vi "Motor Control Message Loop.vi"(8 "error in (no error)":errorcluster, 10 "Data Queue":refnum<queue>, 11 "Message Queues":T1) -> (0 "error out":errorcluster)   [LabVIEW 2016, in "Message Loop Template.lvlib"]
doc: "The message loop subVI to handle messages pertaining to logging data."
uses:
  Message Loop Template.lvlib
  support/Message Queue/All Message Queues.ctl
  support/Message Queue/Message Cluster.ctl
  Motor Control State.ctl
  Motor Control Config.ctl
  Speed and Duration.ctl
  support/Message Queue/Enqueue Message (Single).vi
  <vilib>/Utility/error.llb/Error Cluster From Error Code.vi
  <vilib>/ErrorRing/Error Ring.xnode
  support/Message Queue/Message Queue.lvlib
panel:
  out "Actual Sample Rate":dbl=1000.0 format="%0.2f"
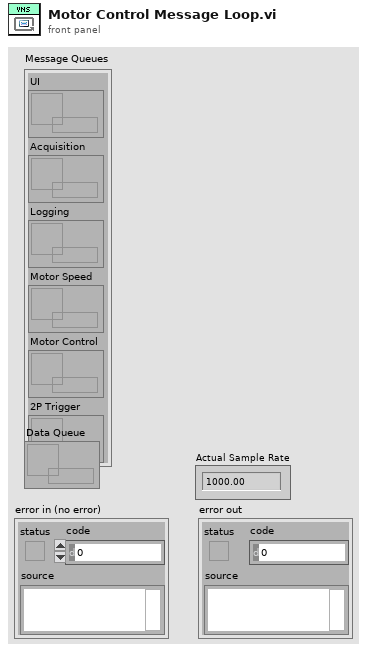
[diagram p1: front panel]
types:
  T1 = typedef "Message Queue.lvlib/All Message Queues.ctl" = cluster{"UI":refnum<queue>, "Acquisition":refnum<queue>, "Logging":refnum<queue>, "Motor Speed":refnum<queue>, "Motor Control":refnum<queue>, "2P Trigger":refnum<queue>}
  T2 = typedef "Message Loop Template.lvlib/Motor Control State.ctl" = enum16{"Idle", "Running"}
  T3 = typedef "Message Loop Template.lvlib/Motor Control Config.ctl" = cluster{"Speed and Duration":T4[]}
  T4 = typedef "Message Loop Template.lvlib/Speed and Duration.ctl" = cluster{"Speed (%)":dbl, "Duration (sec)":dbl}
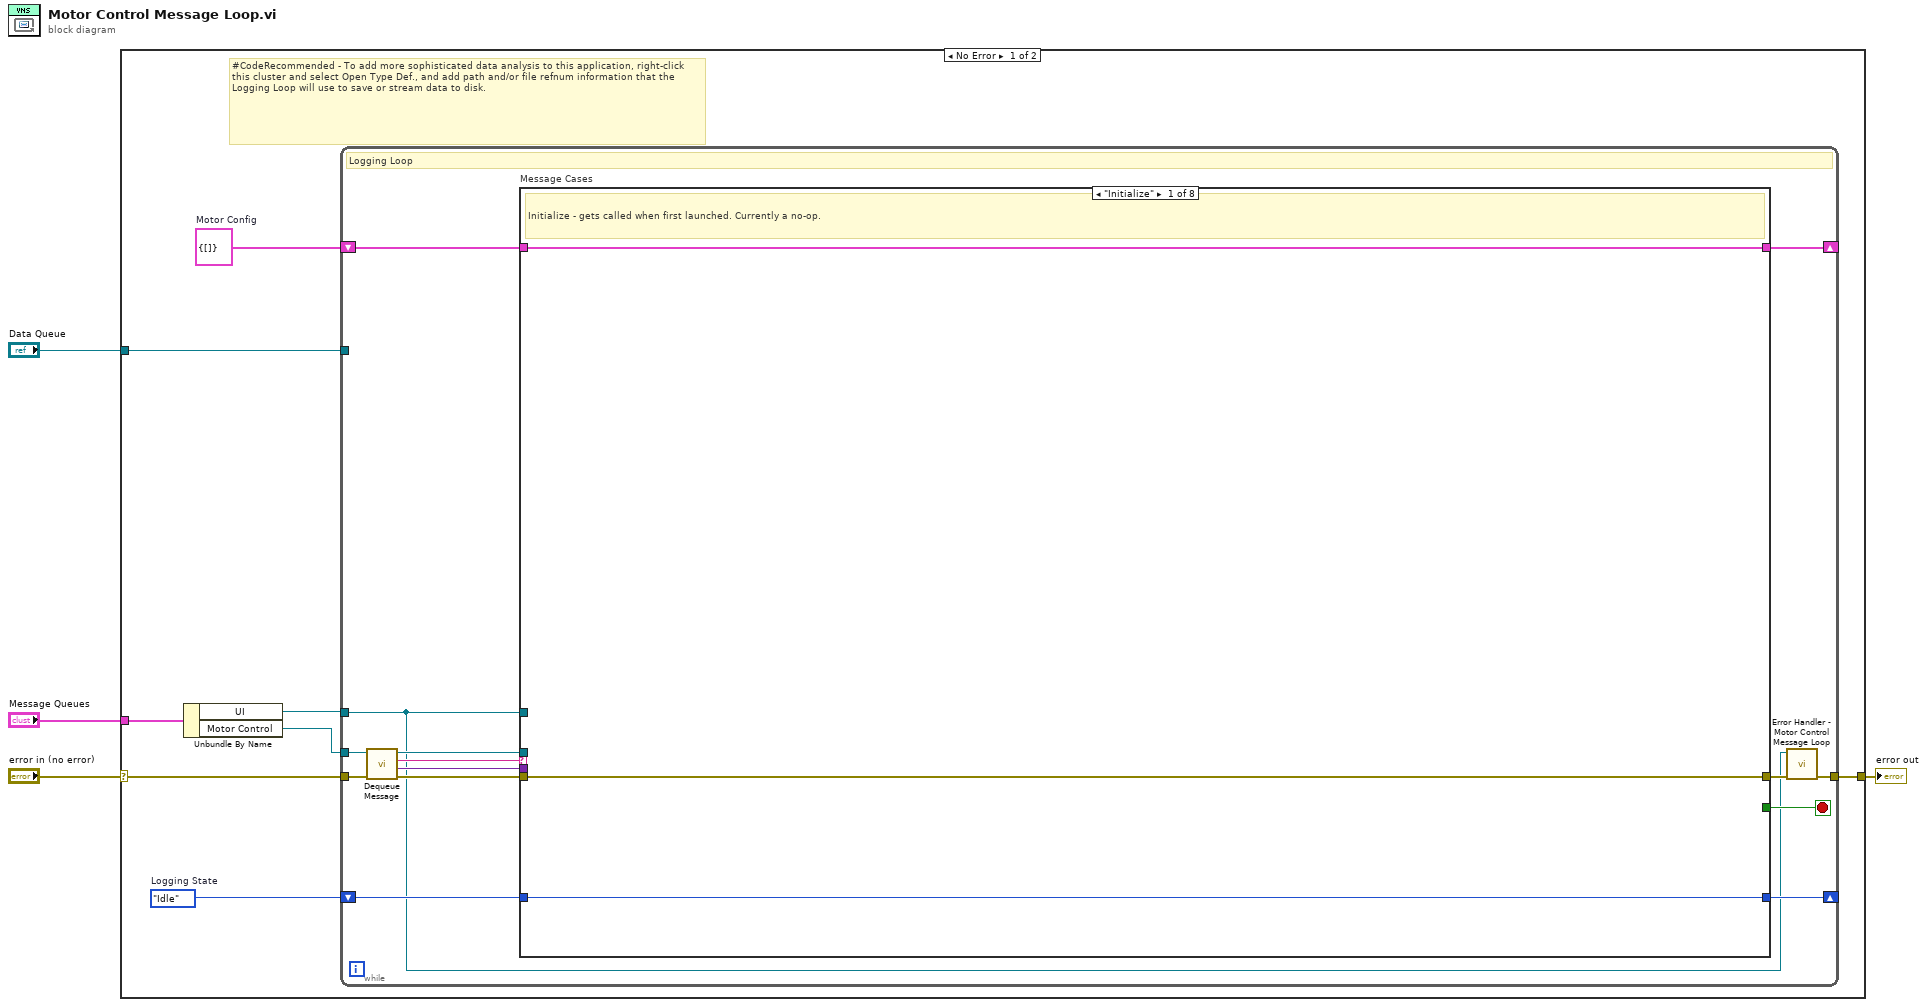
[diagram p0: block diagram]
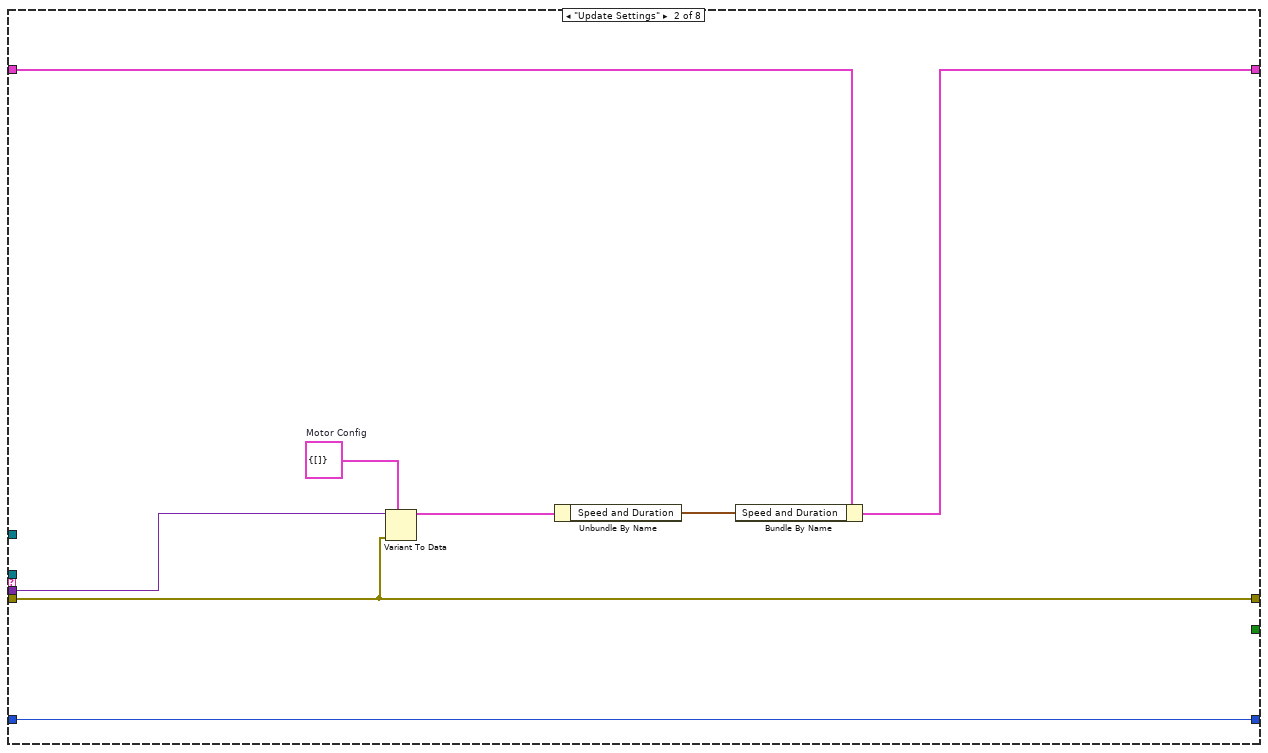
[diagram p2: hidden frame]
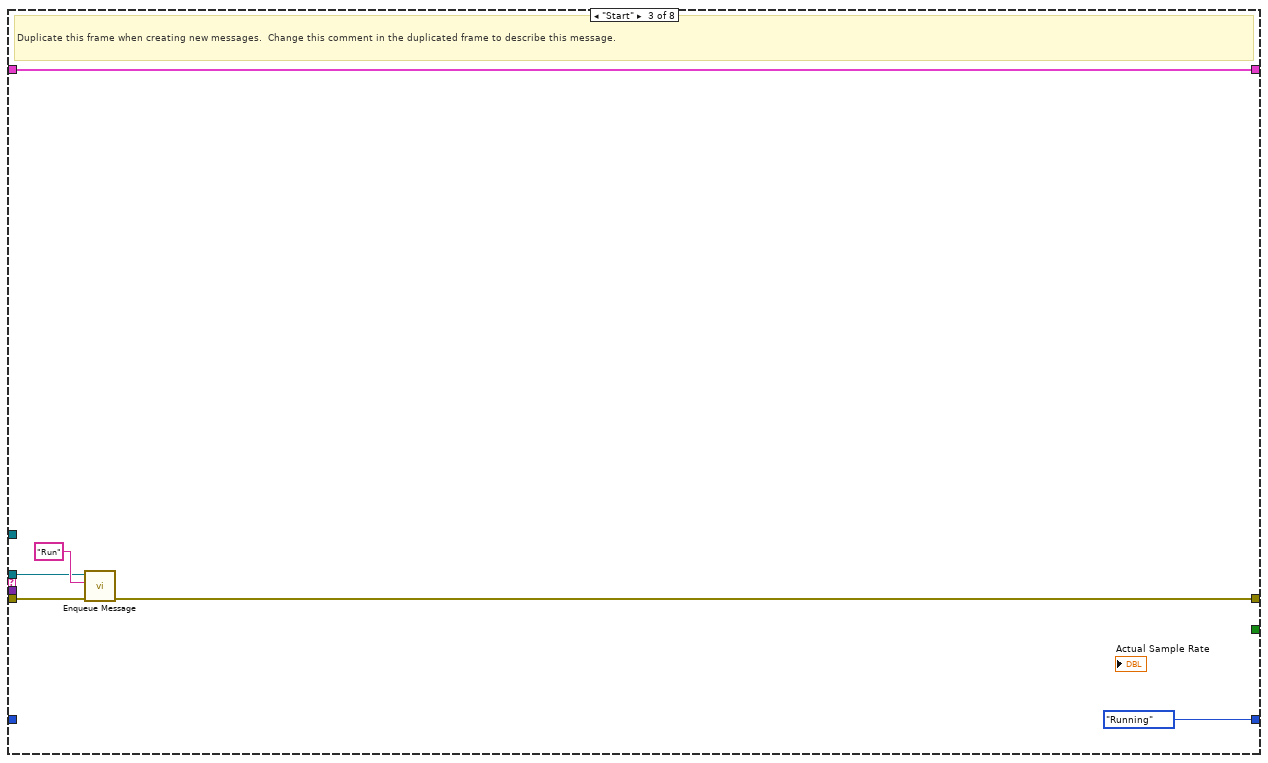
[diagram p3: hidden frame]
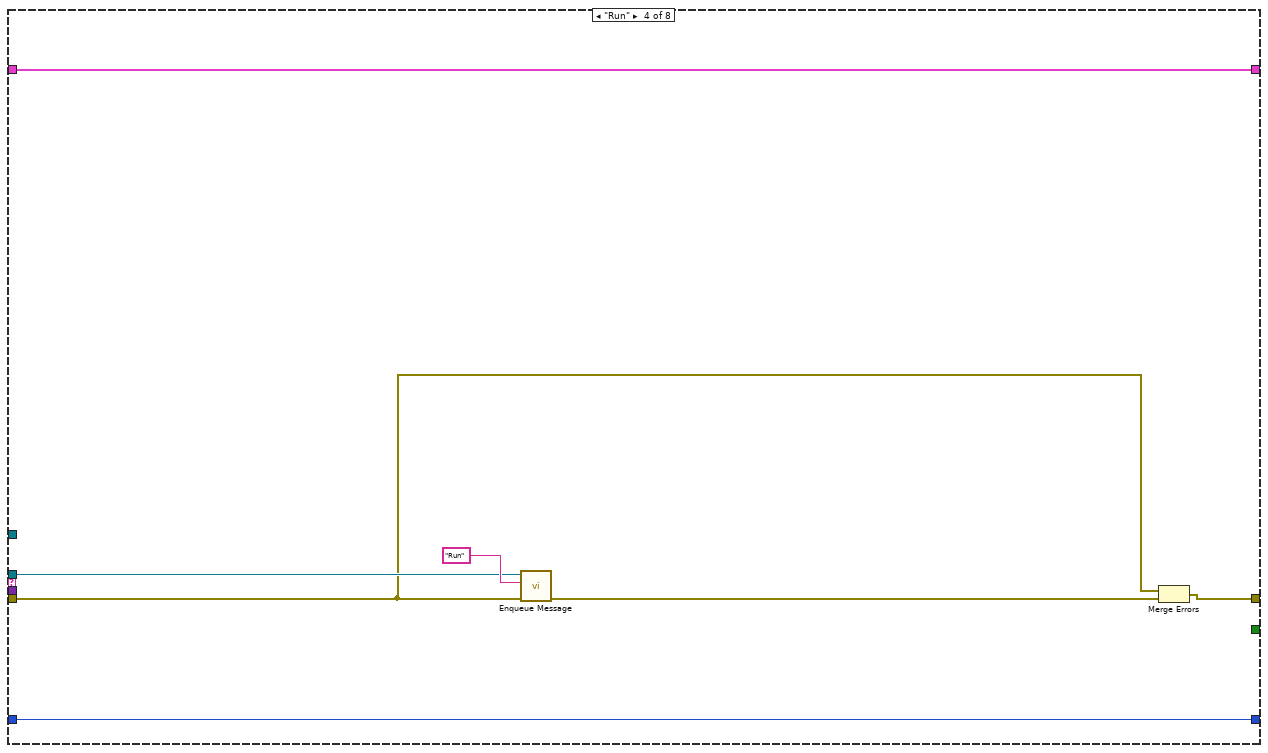
[diagram p4: hidden frame]
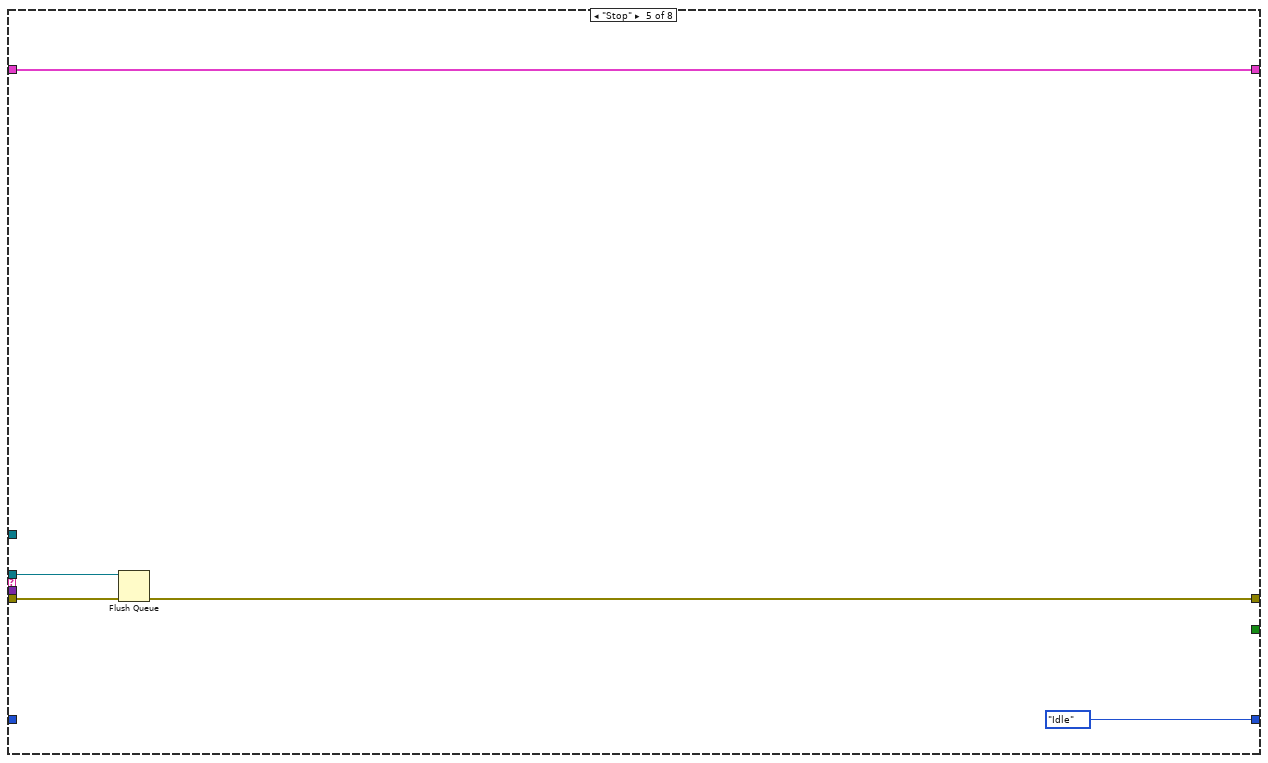
[diagram p5: hidden frame]
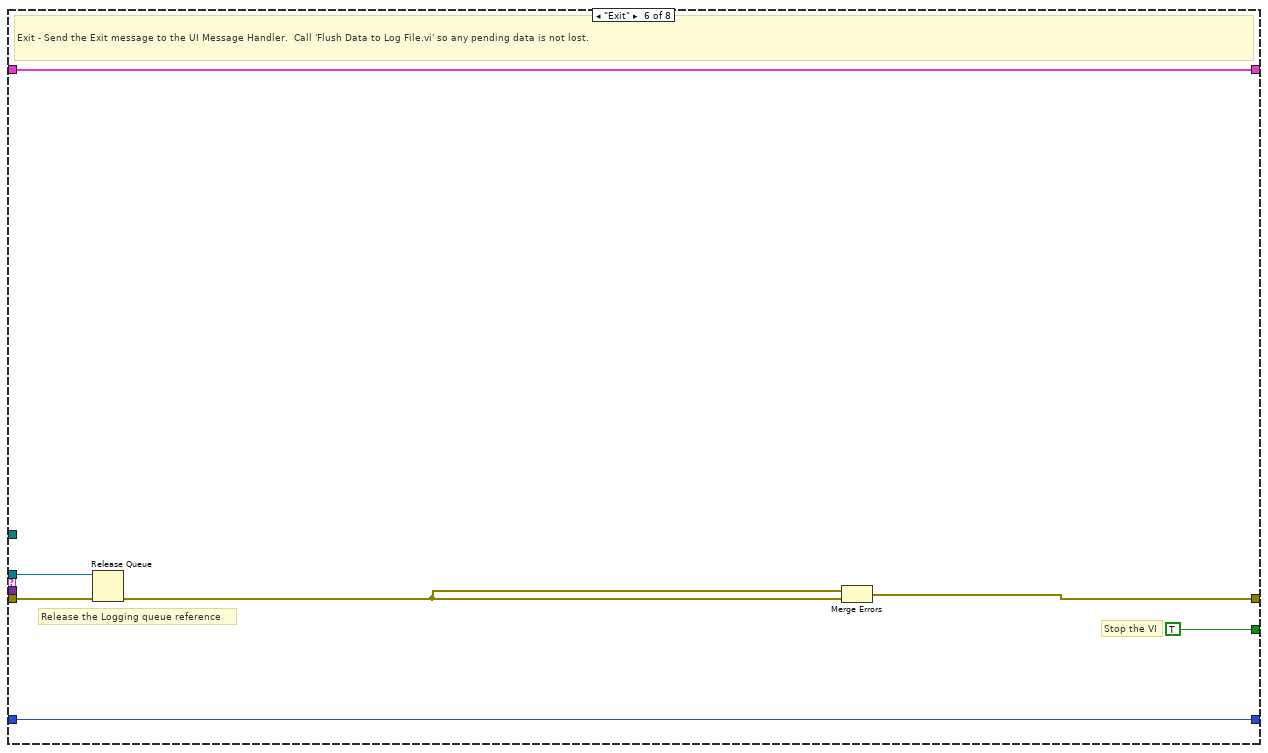
[diagram p6: hidden frame]
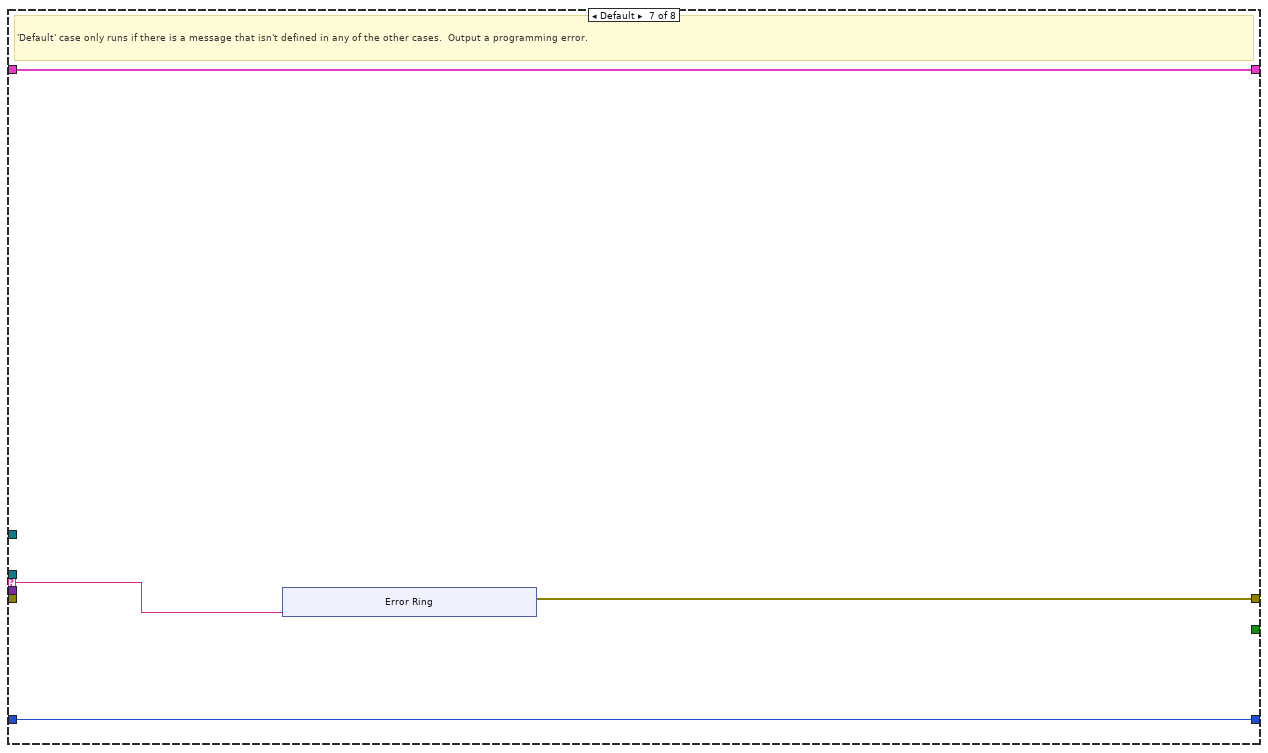
[diagram p7: hidden frame]
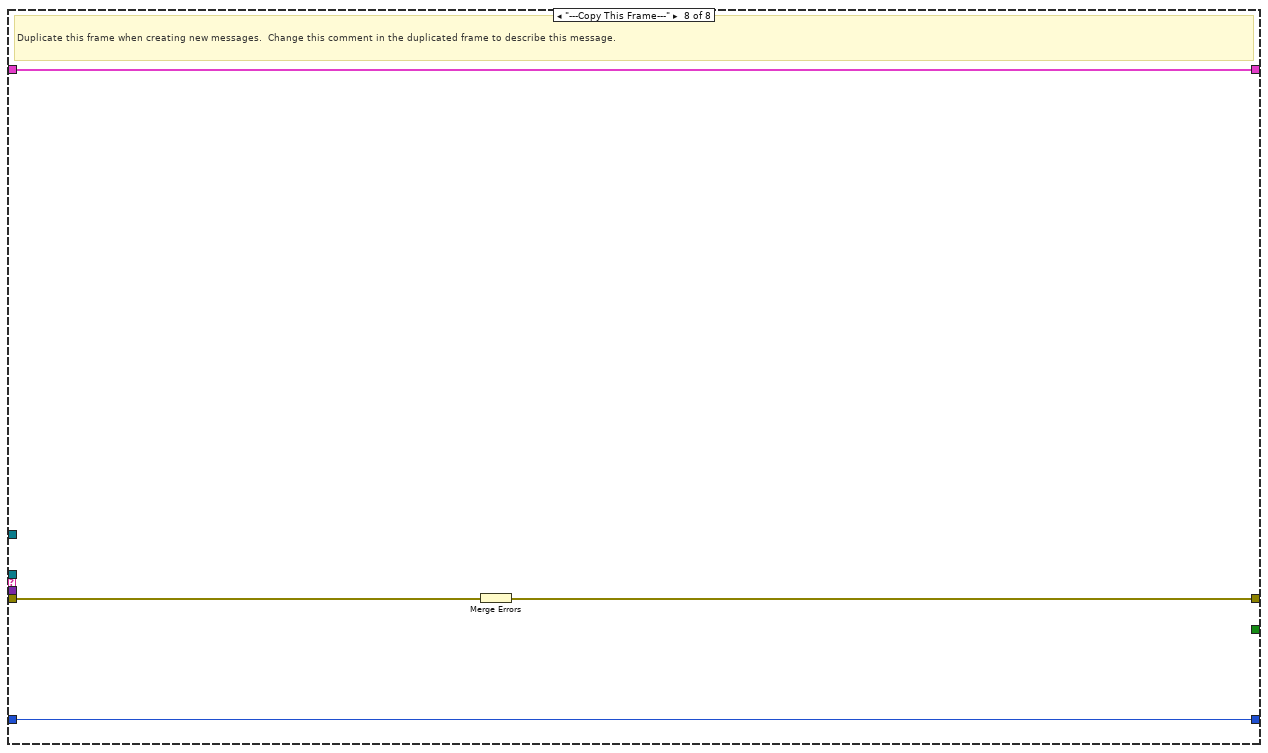
[diagram p8: hidden frame]
diagram:
  n1 = case shown="No Error" "error in (no error)" {
    selector: "error in (no error)" -> [w9 w78]
    tunnel: "Message Queues" -> [w12 _]
    tunnel: [w10 w78] -> w3
    tunnel: "Data Queue" -> [w8 _]
    frame No Error {
      w5 = T3 {"Speed and Duration"=[]}  # Motor Config
      w6 = Motor_Control_State."Idle"  # Logging State
      # "#CodeRecommended - To add more sophisticated data analysis to this application, right-click this cluster and select Open Type Def., and add path and/or file refnum information that the Logging Loop will use to save or stream data to disk."
      n2 = Unbundle By Name(w12) -> ("UI"=w7:refnum<queue>, "Motor Control"=w11:refnum<queue>)
      n3 = while {
        tunnel: w11 -> [w18]
        shift-right: [w25] -> _
        shift-left: w5 -> [w26]
        tunnel: w7 -> [w13]
        tunnel: w8 -> [_]
        shift-right: [w16] -> _
        shift-left: w6 -> [w17]
        tunnel: w9 -> [w23]
        tunnel: [w15] -> w10
        stop <- w24 stop-if-true
        # "Logging Loop"
        n4 = call "Dequeue Message.vi"("error in (no error)"=w23, "Message Queue"=w18) -> ("error out"=w22:errorcluster, "Message Data"=w20:variant, "Message"=w21:string, "dup Message Queue"=w19:refnum<queue>)  [unwired: 6 in]
        n5 = case "Message Cases" shown="\"Initialize\"" w21 {
          selector: w21 -> [_ _ _ _ _ _ w63 _]
          tunnel: w19 -> [_ _ w42 w47 w53 w59 _ _]
          tunnel: w22 -> [w28 w36 w41 w44 w54 w60 _ w77]
          tunnel: [w28 w36 w38 w46 w51 w61 w64 w75] -> w14
          tunnel: w26 -> [w29 w34 w39 w49 w55 w57 w66 w76]
          tunnel: [w29 w33 w39 w49 w55 w57 w66 w76] -> w25
          tunnel: [_ _ _ _ _ TRUE _ _] -> w24
          tunnel: w20 -> [_ w35 _ _ _ _ _ _]
          tunnel: w13 -> [_ _ _ _ _ _ _ _]
          tunnel: w17 -> [w27 w37 _ w50 _ w58 w65 w74]
          tunnel: [w27 w37 Motor_Control_State."Running" ("Logging State") w50 Motor_Control_State."Idle" ("Logging State") w58 w65 w74] -> w16
          frame "Initialize" {
            # "Initialize - gets called when first launched. Currently a no-op."
          }
          frame "Update Settings" {
            w30 = T3 {"Speed and Duration"=[]}  # Motor Config
            n6 = Variant To Data(error in=w36, type=w30, Variant=w35) -> (data=w31:T3)  [unwired: 1 out]
            n7 = Unbundle By Name(w31) -> ("Speed and Duration"=w32:T4[])
            n8 = Bundle By Name(cluster=w34, "Speed and Duration"=w32) -> (w33:T3)
          }
          frame "Start" {
            # "Duplicate this frame when creating new messages.  Change this comment in the duplicated frame to describe this message."
            n9 = call-poly "Enqueue Message.vi"("error in (no error)"=w41, "Message"="Run", "Message Queue"=w42) -> ("error out"=w38:errorcluster)  [unwired: 7 in, 1 out]
          }
          frame "Run" {
            n10 = call-poly "Enqueue Message.vi"("error in (no error)"=w44, "Message"="Run", "Message Queue"=w47) -> ("error out"=w45:errorcluster)  [unwired: 7 in, 1 out]
            n11 = Merge Errors(w44, w45) -> (w46:errorcluster)
          }
          frame "Stop" {
            n12 = Flush Queue(queue=w53, error in (no error)=w54) -> (error out=w51:errorcluster)  [unwired: 2 out]
          }
          frame "Exit" {
            # "Release the Logging queue reference"
            # "Stop the VI"
            # "Exit - Send the Exit message to the UI Message Handler.  Call 'Flush Data to Log File.vi' so any pending data is not lost."
            n13 = Release Queue(queue=w59, error in (no error)=w60) -> (error out=w56:errorcluster)  [unwired: 1 in, 2 out]
            n14 = Merge Errors(w56, w56) -> (w61:errorcluster)
          }
          frame Default {
            # "'Default' case only runs if there is a message that isn't defined in any of the other cases.  Output a programming error."
            n15 = xnode "Error Ring"("parameter 0"=w63) -> ("error out"=w64:errorcluster)
          }
          frame "---Copy This Frame---" {
            # "Duplicate this frame when creating new messages.  Change this comment in the duplicated frame to describe this message."
            n16 = Merge Errors(w77) -> (w75:errorcluster)
          }
        }
        n17 = call "Error Handler - Motor Control Message Loop.vi"("error in (no error)"=w14, "Message Queue"=w13) -> ("dup error in"=w15:errorcluster)  [unwired: 8 in, 1 out]
      }
    }
    frame Error {
    }
  }
  "error out" <- w3
